vi "SetCameraParameter.vi"(2 "error in":errorcluster, 3 "相机品牌为Basler?":bool, 4 "Exposure time":i64, 5 "Session In":T1="cam0") -> (0 "error out":errorcluster, 1 "Session Out":T1)   [LabVIEW 2014]
uses:
  <vilib>/userdefined/High Color/IMAQdx.ctl
  <resource>/objmgr/imaqdx.rc
panel:
  # "200"
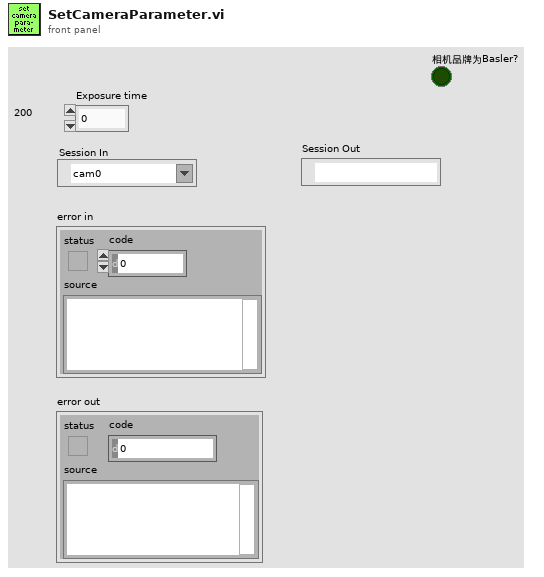
[diagram p1: front panel]
types:
  T1 = typedef "IMAQdx.ctl" = refnum<k21>
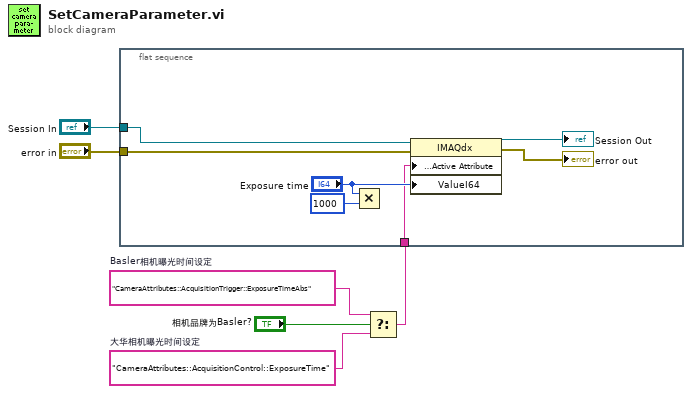
[diagram p0: block diagram]
diagram:
  w4 = "CameraAttributes::AcquisitionTrigger::ExposureTimeAbs"  # Basler相机曝光时间设定
  w3 = "CameraAttributes::AcquisitionControl::ExposureTime"  # 大华相机曝光时间设定
  n1 = flat-sequence {
    tunnel: "error in" -> [w10]
    tunnel: "Session In" -> [w11]
    tunnel: w1 -> [w7]
    frame #0 {
      n2 = Multiply(x="Exposure time", y=i64 1000) -> ()  [unwired: 1 out]
      n3 = property on="Property Node" class="IMAQdx"(reference=w11, error in=w10, "Camera Attributes:Active Attribute"=w7, "ValueI64"="Exposure time") -> (reference out=→"Session Out":T1, error out=→"error out":errorcluster)
    }
  }
  n4 = Select(t=w4, s="相机品牌为Basler?", f=w3) -> (s? t:f=w1:string)
